vi "field-global.vi"() -> ()   [LabVIEW 2013]
panel:
  in  "Field Array":dbl[](array[numeric])
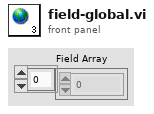
[diagram p1: front panel]
diagram:
